vi "Process.vi"(8 "error in (no error)":errorcluster, 10 "Json Data":string, 11 "InferenceMock in":refnum<class "InferenceMock.lvclass">) -> (0 "error out":errorcluster, 3 "InferenceMock out":refnum<class "InferenceMock.lvclass">)   [LabVIEW 2019, in "InferenceMock.lvlib" / "InferenceMock.lvclass"]
uses:
  InferenceMock.lvclass
  C:/Repos/Demo/Actors/AI Inference/Inference/Inference/Inference.lvclass
  InferenceMock.lvclass/InferenceMock.ctl
  Models/InferenceDataModel.ctl
  Models/InferenceResultsModel.ctl
  6e2e6973-7a55-4536-a053-2c97fbf8cf51.vi
  f1eb05cb-6019-49f4-a206-3f5b9e028e3f.vi
  <vilib>/JDP Science/JSONtext/JSON text to Variant.vi
  <vilib>/JDP Science/JSONtext/Variant to JSON Text.vi
  <vilib>/JDP Science/JSONtext/LVClass Serializer/JSONtext LVClass Serializer.lvclass
  Inference/Inference/Inference.lvclass
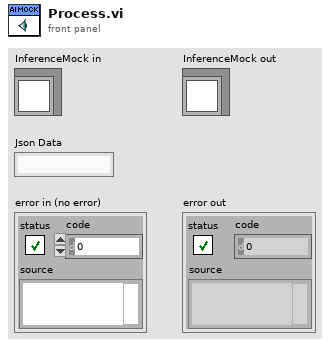
[diagram p1: front panel]
types:
  T1 = typedef "InferenceResultsModel.ctl" = cluster{"guid":string, "results":cluster{"pass":bool, "class":string}[], "time":dbl}
  T2 = typedef "InferenceDataModel.ctl" = cluster{"guid":string, "images":string[]}
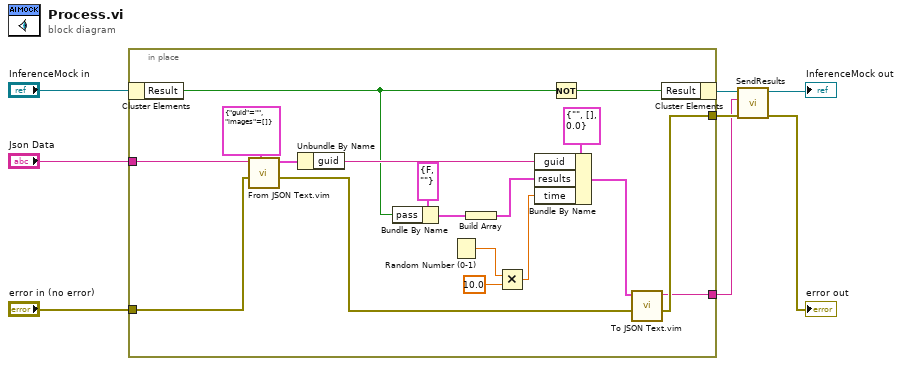
[diagram p0: block diagram]
diagram:
  n1 = in-place {
    in-place-border: "error in (no error)" -> [w23]
    in-place-border: "Json Data" -> [w25]
    in-place-border: [w13] -> w2
    in-place-border: [w12] -> w1
    n2 = in-place-cluster #1("InferenceMock in") -> ("Result"=w18:bool)
    n3 = call "From JSON Text.vim"("Data Type and Default Value"=T2 {"guid"="", "images"=[]} ("Data"), "error in (no error)"=w23, "JSON"=w25) -> ("error out"=w14:errorcluster, "Data out"=w22:T2)  [unwired: 7 in]
    n4 = Unbundle By Name(w22) -> ("guid"=w20:string)
    n5 = Bundle By Name(cluster=cluster{"pass":bool, "class":string} {"pass"=FALSE, "class"=""} ("results"), "pass"=w18) -> (w17:cluster{"pass":bool, "class":string})
    n6 = Random Number (0-1)() -> (number: 0 to 1=w11:dbl)
    n7 = Build Array(w17) -> (w16:cluster{"pass":bool, "class":string}[])
    n8 = Multiply(x=w11, y=10.0) -> (x*y=w9:dbl)
    n9 = Bundle By Name(cluster=T1 {"guid"="", "results"=[], "time"=0.0} ("data"), "guid"=w20, "results"=w16, "time"=w9) -> (w15:T1)
    n10 = Not(x=w18) -> (.not. x?=w26:bool)
    n11 = call "To JSON Text.vim"("error in (no error)"=w14, "Anything"=w15) -> ("error out"=w13:errorcluster, "<JSON>"=w12:string)  [unwired: 8 in]
    n12 = in-place-cluster #1("Result"=w26) -> (w5:refnum<class "InferenceMock.lvclass">)
  }
  n13 = call "SendResults.vi"("error in (no error)"=w2, "Result Json"=w1, "Inference in"=w5) -> ("error out"=→"error out":errorcluster, "Inference out"=→"InferenceMock out":refnum<class "InferenceMock.lvclass">)  [unwired: 7 in]
